vi "Shutdown.vi"(8 "error in":errorcluster, 11 "Oscilloscope in":refnum<class "Oscilloscope.lvclass">) -> (0 "error out":errorcluster, 3 "Oscilloscope out":refnum<class "Oscilloscope.lvclass">)   [LabVIEW 2019, in "Oscilloscope.lvlib" / "Oscilloscope.lvclass"]
uses:
  Oscilloscope.lvclass
  builds/Instruments/Instruments.lvlibp/Library/Instruments.lvclass
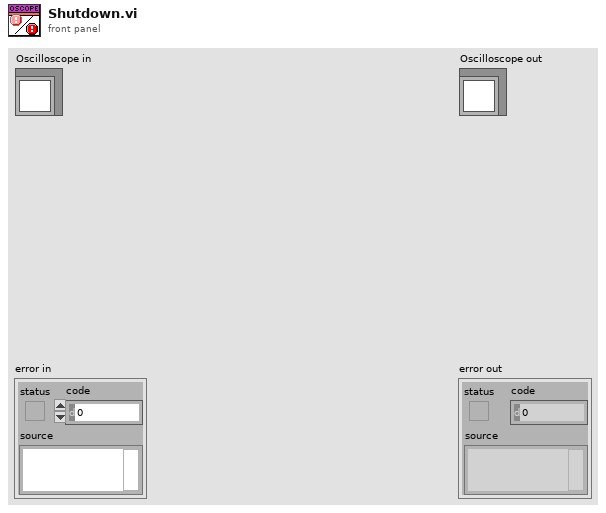
[diagram p1: front panel]
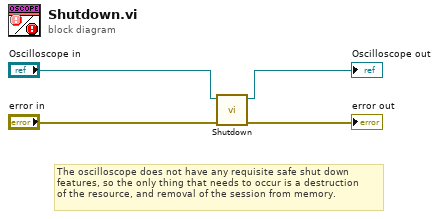
[diagram p0: block diagram]
diagram:
  # "The oscilloscope does not have any requisite safe shut down \nfeatures, so the only thing that needs to occur is a destruction\nof the resource, and removal of the session from memory."
  n1 = call-parent "Shutdown.vi"("error in"="error in", "Instruments in"="Oscilloscope in") -> ("error out"=→"error out":errorcluster, "Instruments out"=→"Oscilloscope out":refnum<class "Oscilloscope.lvclass">)  [unwired: 8 in]
